vi "Delete row(s).vi"(8 "error in (no error)":errorcluster, 10 "Row Indices":i32[](array[numeric]), 11 "MulColLBTable.lvclass":refnum<class "MulColLBTable.lvclass">) -> (0 "error out":errorcluster, 3 "MulColLBTable.lvclass 2":refnum<class "MulColLBTable.lvclass">)   [LabVIEW 2020, in "MulColLBTable.lvclass"]
uses:
  MulColLBTable.lvclass
  MulColLBTable.lvclass/MulColLBTable.ctl
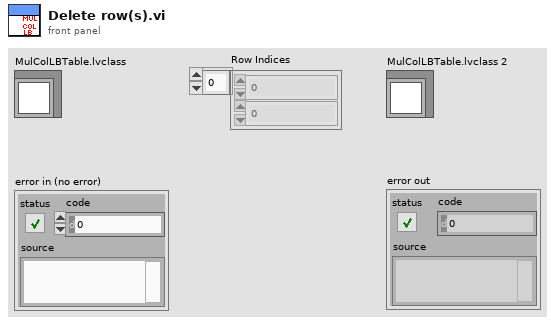
[diagram p1: front panel]
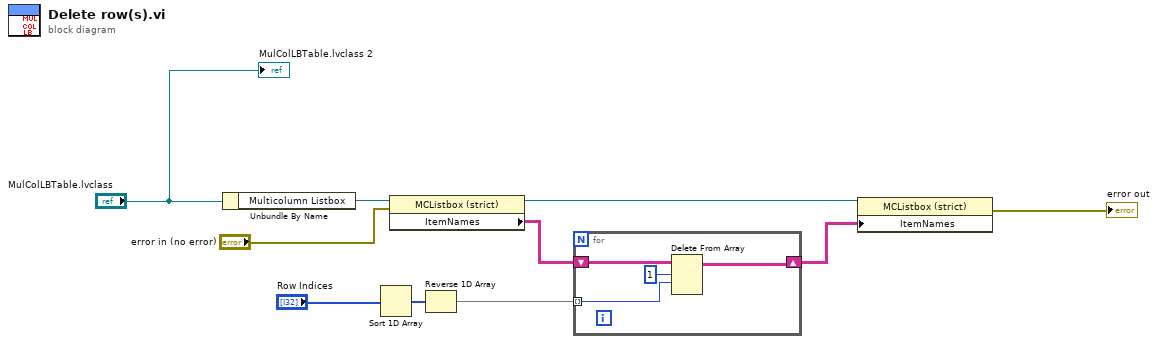
[diagram p0: block diagram]
diagram:
  n1 = Unbundle By Name("MulColLBTable.lvclass") -> ("Multicolumn Listbox"=w9:refnum<vi>)
  n2 = Sort 1D Array(array="Row Indices") -> (sorted array=w3:i32[])
  n3 = property class="MCListbox (strict)"(reference=w9, error in="error in (no error)") -> (reference out=w8:refnum<vi>, "ItemNames"=w5:string[][])  [unwired: 1 out]
  n4 = Reverse 1D Array(array=w3) -> (reversed array=w1:i32[])
  n5 = for {
    shift-right: [w13] -> w4
    shift-left: w5 -> [w14]
    tunnel: w1 -> [w11] mode=indexing
    n6 = Delete From Array(array=w14, length=1, index (row)=w11) -> (array with subset deleted=w13:string[][])  [unwired: 1 in, 1 out]
  }
  n7 = property class="MCListbox (strict)"(reference=w8, "ItemNames"=w4) -> (error out=→"error out":errorcluster)  [unwired: 1 in, 1 out]
  "MulColLBTable.lvclass 2" <- "MulColLBTable.lvclass"
